vi "Send command Set Port.vi"(7 "Marca":string, 8 "error in (no error)":errorcluster, 9 "Valor HEX":string, 10 "Puerto":string, 11 "Serial Device in":refnum<class "Serial Device.lvclass">) -> (0 "error out":errorcluster, 1 "Command":string, 2 "Expected response":string, 3 "Serial Device out":refnum<class "Serial Device.lvclass">)   [LabVIEW 2020, in "Serial Device.lvclass"]
uses:
  Serial Device.lvclass
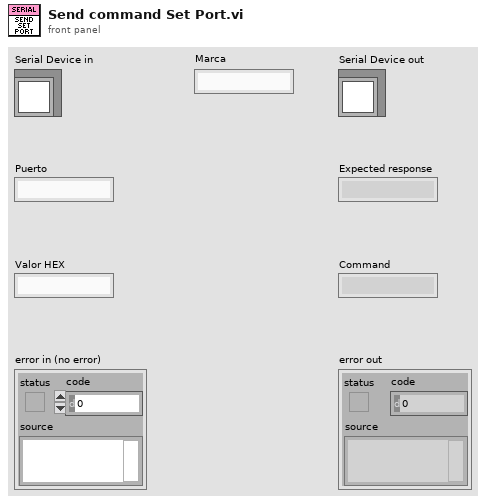
[diagram p1: front panel]
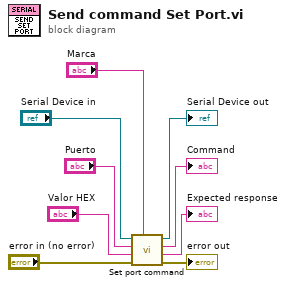
[diagram p0: block diagram]
diagram:
  n1 = call-dynamic "Set port command.vi"("Marca"="Marca", "error in (no error)"="error in (no error)", "Valor HEX"="Valor HEX", "Puerto"="Puerto", "Serial Device in"="Serial Device in") -> ("error out"=→"error out":errorcluster, "Expected response"=→"Expected response":string, "Command"=→"Command":string, "Serial Device out"=→"Serial Device out":refnum<class "Serial Device.lvclass">)  [unwired: 3 in]
